vi "Run Protocol.vi"(8 "error in (no error)":errorcluster, 11 "Time Protocol in":refnum<class "Time Protocol.lvclass">) -> (0 "error out":errorcluster, 3 "Time Protocol out":refnum<class "Time Protocol.lvclass">)   [LabVIEW 2012, in "Time Protocol Actor.lvlib" / "Time Protocol.lvclass"]
uses:
  Time Protocol.lvclass
  Time Protocol.lvclass/Time Protocol.ctl
  Read DVR.vi
  Read History.vi
  Read Code.vi
  Read State.vi
  <vilib>/Utility/file.llb/Read From Spreadsheet File (string).vi
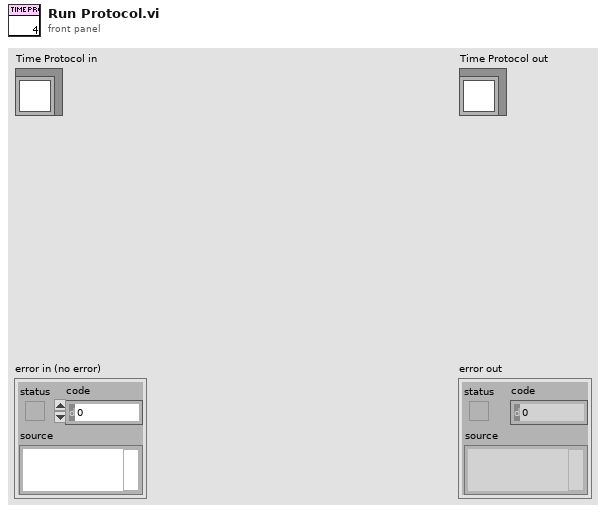
[diagram p1: front panel]
types:
  T1 = enum32{"Pause Button", "Play Button", "Media Stop Button"}
  T2 = cluster{"Name":string, "Value":dbl, "Setpoint":dbl, "Output":dbl}[]
  T3 = cluster{"Name":string, "Value":dbl, "Setpoint":dbl, "Output":dbl}
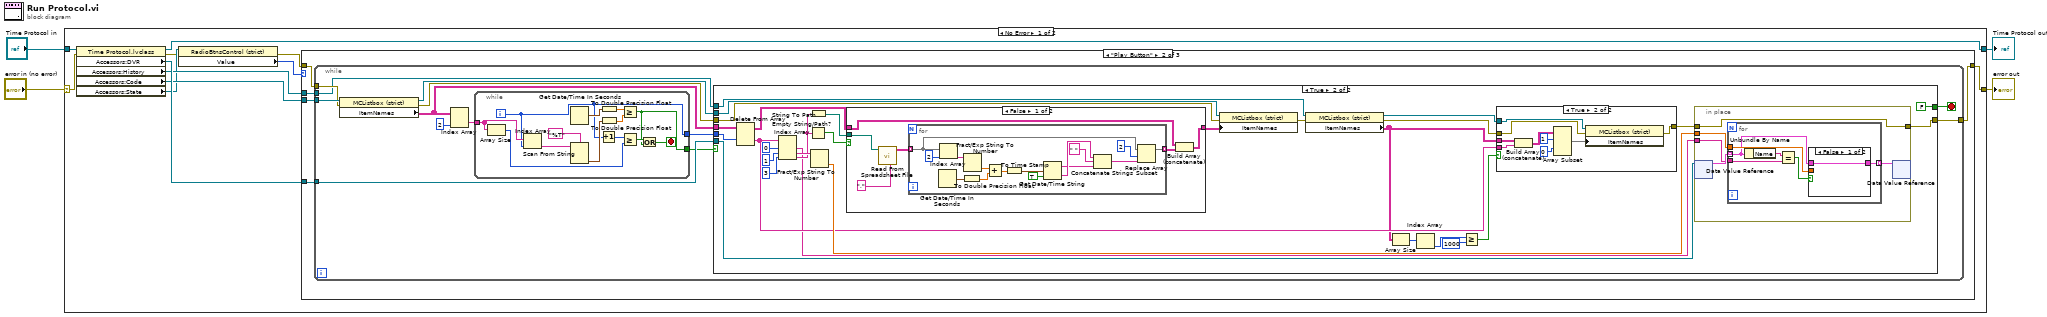
[diagram p0: block diagram]
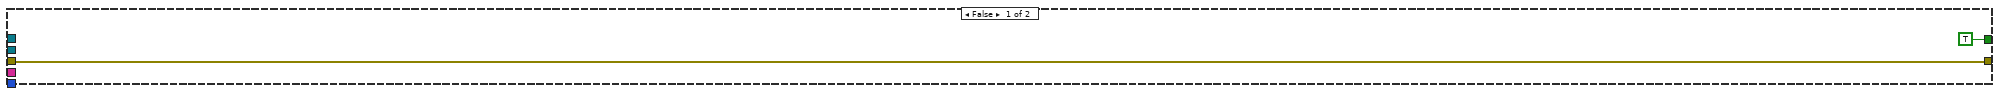
[diagram p3: hidden frame]
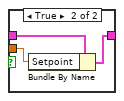
[diagram p4: hidden frame]
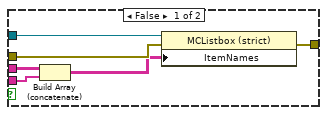
[diagram p5: hidden frame]
diagram:
  n1 = case shown="No Error" "error in (no error)" {
    selector: "error in (no error)" -> [w6 w133]
    tunnel: [w5 w133] -> w3
    tunnel: [w13 w132] -> w1
    tunnel: "Time Protocol in" -> [w12 w132]
    frame No Error {
      n2 = property class="Time Protocol.lvclass"(reference=w12, error in=w6) -> (reference out=w13:refnum<class "Time Protocol.lvclass">, error out=w7:errorcluster, "Accessors:DVR"=w11:refnum<data-value>, "Accessors:History"=w10:refnum<vi>, "Accessors:Code"=w9:refnum<vi>, "Accessors:State"=w8:refnum<vi>)
      n3 = property class="RadioBtnsControl (strict)"(reference=w8, error in=w7) -> (error out=w15:errorcluster, "Value"=w14:T1)  [unwired: 1 out]
      n4 = case shown="\"Play Button\"" w14 {
        tunnel: w11 -> [_ w21 _]
        tunnel: [w16 w18 w131] -> w5
        tunnel: w9 -> [_ w20 _]
        tunnel: w15 -> [w16 w19 w131]
        tunnel: w10 -> [_ w17 _]
        frame "Pause Button", Default {
        }
        frame "Play Button" {
          n5 = while {
            tunnel: w21 -> [w34]
            tunnel: w20 -> [w33]
            tunnel: w19 -> [w32]
            tunnel: [w26] -> w18
            tunnel: w17 -> [w23]
            stop <- w22 stop-if-true
            n6 = property class="MCListbox (strict)"(reference=w33, error in=w32) -> (reference out=w27:refnum<vi>, error out=w28:errorcluster, "ItemNames"=w29:string[][])
            n7 = Index Array(array=w29, index (col)=2 ("disabled index (col)")) -> (element=w30:string[])  [unwired: 1 in]
            n8 = while {
              tunnel: w30 -> [w123]
              tunnel: [w119] -> w25
              tunnel: [w118] -> w24
              i -> [w119]
              stop <- w120 stop-if-true
              n9 = Array Size(array=w123) -> (size(s)=w124:i32)
              n10 = Index Array(array=w123, index=w119) -> (element=w122:string)
              n11 = Get Date/Time In Seconds() -> (seconds since 1Jan1904=w128:timestamp)
              n12 = Scan From String(format string="%T", input string=w122) -> (output 1=w129:timestamp)  [unwired: 3 in, 3 out]
              n13 = Increment(x=w119) -> (x+1=w125:i32)
              n14 = To Double Precision Float(number=w128) -> (double precision float=w126:dbl)
              n15 = To Double Precision Float(number=w129) -> (double precision float=w127:dbl)
              n16 = Greater Or Equal?(x=w126, y=w127) -> (x >= y?=w118:bool)
              n17 = Greater Or Equal?(x=w125, y=w124) -> (x >= y?=w121:bool)
              n18 = Or(x=w121, y=w118) -> (x .or. y?=w120:bool)
            }
            n19 = case shown="True" w24 {
              tunnel: w34 -> [_ w65]
              tunnel: w29 -> [_ w64]
              tunnel: w28 -> [w36 w51]
              tunnel: w27 -> [_ w57]
              tunnel: [w36 w58] -> w26
              tunnel: w25 -> [_ w56]
              tunnel: w23 -> [_ w53]
              tunnel: [TRUE FALSE] -> w22
              frame False {
              }
              frame True {
                n20 = Delete From Array(array=w64, index (row)=w56) -> (deleted portion=w49:string[], array with subset deleted=w44:string[][])  [unwired: 2 in]
                n21 = Index Array(array=w49, index #1=0 ("index"), index #2=1 ("index"), index #3=3 ("index")) -> (element #1=w37:string, element #2=w60:string, element #3=w46:string)
                n22 = Empty String/Path?(string/path=w46) -> (empty?=w47:bool)
                n23 = String To Path(string=w46) -> (path=w45:path)
                n24 = Fract/Exp String To Number(string=w60) -> (number=w59:dbl)  [unwired: 3 in, 1 out]
                n25 = case shown="False" w47 {
                  tunnel: w45 -> [w101 _]
                  tunnel: w44 -> [w99 w117]
                  tunnel: [w97 w117] -> w43
                  frame False {
                    n26 = call-poly <vilib>:"Read From Spreadsheet File.vi"("delimiter (\\t)"="," ("delimiter (\\t)"), "file path (dialog if empty)"=w101) -> ("all rows"=w100:string[][])  [unwired: 5 in, 4 out]
                    n27 = for {
                      tunnel: w100 -> [w111] mode=indexing
                      tunnel: [w108] -> w98 mode=indexing
                      n28 = Get Date/Time In Seconds() -> (seconds since 1Jan1904=w115:timestamp)
                      n29 = Index Array(array=w111, index=2) -> (element=w114:string)
                      n30 = To Double Precision Float(number=w115) -> (double precision float=w112:dbl)
                      n31 = Fract/Exp String To Number(string=w114) -> (number=w113:dbl)  [unwired: 3 in, 1 out]
                      n32 = Add(x=w113, y=w112) -> (x+y=w109:dbl)
                      n33 = To Time Stamp(1:w109) -> (0:w104:timestamp)
                      n34 = Get Date/Time String(seconds (now)=w104, want seconds? (F)=TRUE) -> (date string=w106:string, time string=w107:string)  [unwired: 1 in]
                      n35 = Concatenate Strings(w107, " " ("string"), w106) -> (w103:string)
                      n36 = Replace Array Subset(array=w111, new element=w103, index=2) -> (w108:string[])
                    }
                    n37 = Build Array (concatenate)(w99, w98) -> (w97:string[][])
                  }
                  frame True {
                  }
                }
                n38 = property class="MCListbox (strict)"(reference=w57, error in=w51, "ItemNames"=w43) -> (error out=w52:errorcluster)  [unwired: 1 out]
                n39 = property class="MCListbox (strict)"(reference=w53, error in=w52) -> (reference out=w54:refnum<vi>, error out=w55:errorcluster, "ItemNames"=w42:string[][])
                n40 = Array Size(array=w42) -> (size(s)=w41:i32[])
                n41 = Index Array(array=w41) -> (element=w40:i32)  [unwired: 1 in]
                n42 = Greater Or Equal?(x=w40, y=1000) -> (x >= y?=w38:bool)
                n43 = case shown="True" w38 {
                  tunnel: w55 -> [w86 w95]
                  tunnel: w54 -> [w85 w94]
                  tunnel: [w84 w93] -> w50
                  tunnel: w42 -> [w83 w92]
                  tunnel: w49 -> [w82 w91]
                  frame False {
                    n44 = Build Array (concatenate)(w83, w82) -> (w81:string[][])
                    n45 = property class="MCListbox (strict)"(reference=w85, error in=w86, "ItemNames"=w81) -> (error out=w84:errorcluster)  [unwired: 1 out]
                  }
                  frame True {
                    n46 = Build Array (concatenate)(w92, w91) -> (w90:string[][])
                    n47 = Array Subset(array=w90, index (row)=1 ("index"), index (col)=0 ("index")) -> (w87:string[][])  [unwired: 2 in]
                    n48 = property class="MCListbox (strict)"(reference=w94, error in=w95, "ItemNames"=w87) -> (error out=w93:errorcluster)  [unwired: 1 out]
                  }
                }
                n49 = in-place {
                  in-place-border: [w70] -> w58
                  in-place-border: w50 -> [w70]
                  in-place-border: w59 -> [w67]
                  in-place-border: w37 -> [w66]
                  n50 = in-place-dvr #1(w65) -> (w69:T2)  [unwired: 1 out]
                  n51 = for {
                    tunnel: w69 -> [w74] mode=indexing
                    tunnel: [w76] -> w68 mode=indexing
                    tunnel: w67 -> [w75]
                    tunnel: w66 -> [w72]
                    n52 = Unbundle By Name(w74) -> ("Name"=w73:string)
                    n53 = Equal?(x=w73, y=w72) -> (x = y?=w71:bool)
                    n54 = case shown="False" w71 {
                      tunnel: [w77 w80] -> w76
                      tunnel: w75 -> [_ w79]
                      tunnel: w74 -> [w77 w78]
                      frame False {
                      }
                      frame True {
                        n55 = Bundle By Name(cluster=w78, "Setpoint"=w79) -> (w80:T3)
                      }
                    }
                  }
                  n56 = in-place-dvr #1(w68) -> ()  [unwired: 2 out]
                }
              }
            }
          }
        }
        frame "Media Stop Button" {
        }
      }
    }
    frame Error {
    }
  }
  "error out" <- w3
  "Time Protocol out" <- w1
